vi "Load Test Data.vi"(8 "error in (no error)":errorcluster, 9 "To":timestamp, 10 "From":timestamp, 11 "Access in":refnum<class "Access.lvclass">) -> (0 "error out":errorcluster, 2 "Test Data Out":string[][](array[string]), 3 "Access out":refnum<class "Access.lvclass">)   [LabVIEW 2016, in "Database.lvlib" / "Access.lvclass"]
uses:
  Access.lvclass
  Access.lvclass/Access.ctl
  <vilib>/addons/database/Connection.llb/Conn Execute.vi
  <vilib>/addons/database/Recordset.llb/Rec Fetch Recordset Data (R).vi
  <vilib>/addons/database/Recordset.llb/Rec Destroy - Connection.vi
  <vilib>/addons/database/NI_Database_API.lvlib
  User Interface/User Interface.lvlib
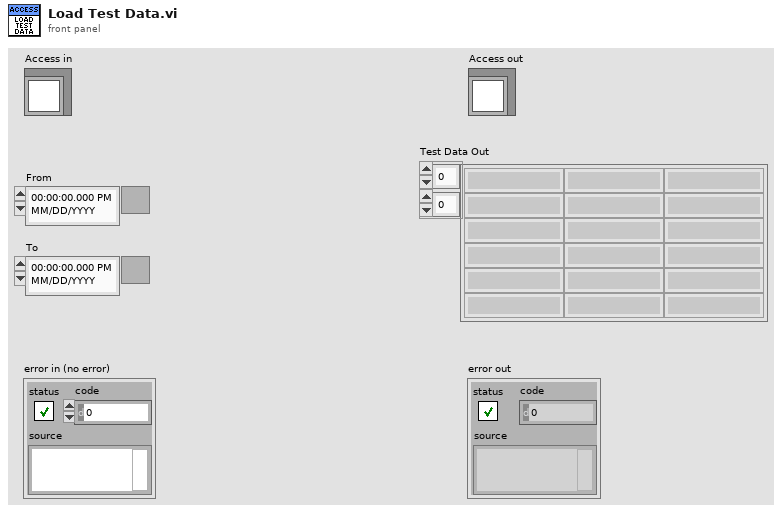
[diagram p1: front panel]
types:
  T1 = typedef "Database.lvlib/DB.lvclass/Column_info.ctl" = cluster{"Authentication":T2[], "Instr_Configuration":T2[], "Recipe":T2[], "Test_data":T2[]}
  T2 = typedef "NI_Database_API.lvlib/DB Tools Column Info.ctl" = cluster{"column name":string, "data type":T3, "size":i32, "allow null?":bool}
  T3 = typedef "NI_Database_API.lvlib/DB Tools DataTypes.ctl" = enum16{"String", "Long (I32)", "Single (SGL)", "Double (DBL)", "Date/Time", "Binary"}
  T4 = typedef "Database.lvlib/DB.lvclass/Table_info.ctl" = cluster{"Authentication":string, "Instr_Configuration":string, "Recipe":string, "Test_data":string}
  T5 = typedef "NI_Database_API.lvlib/Conn ObjectReference.ctl" = refnum<k1>
  T6 = typedef "NI_Database_API.lvlib/Rec ObjectReference.ctl" = refnum<k1>
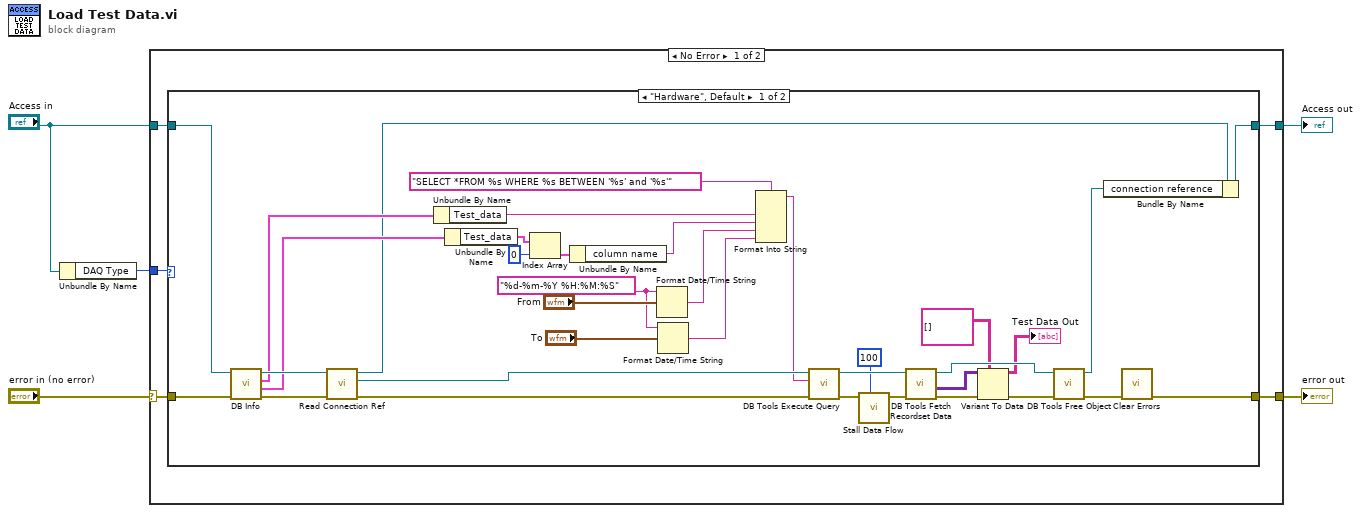
[diagram p0: block diagram]
diagram:
  n1 = Unbundle By Name("Access in") -> ("DAQ Type"=w1:enum16{"Hardware", "Simulation"})
  n2 = case shown="No Error" "error in (no error)" {
    selector: "error in (no error)" -> [w10 w48]
    tunnel: [w8 w49] -> w4
    tunnel: "Access in" -> [w9 w49]
    tunnel: [w7 w48] -> w3
    tunnel: w1 -> [w6 _]
    frame No Error {
      n3 = case shown="\"Hardware\", Default" w6 {
        tunnel: w10 -> [w45 w46]
        tunnel: w9 -> [w12 w47]
        tunnel: [w38 w47] -> w8
        tunnel: [w15 w46] -> w7
        frame "Hardware", Default {
          w21 = "%d-%m-%Y %H:%M:%S" ("time format string (%c)")
          n4 = call-dynamic "DB Info.vi"("error in (no error)"=w45, "Access in"=w12) -> ("error out"=w44:errorcluster, "Column_info"=w30:T1, "Table_info"=w33:T4, "Access out"=w43:refnum<class "Access.lvclass">)  [unwired: 6 in]
          n5 = call-dynamic "Read Connection Ref.vi"("error in (no error)"=w44, "Access in"=w43) -> ("error out"=w42:errorcluster, "connection reference"=w35:T5, "Access out"=w11:refnum<class "Access.lvclass">)  [unwired: 7 in]
          n6 = Unbundle By Name(w33) -> ("Test_data"=w31:string)
          n7 = Unbundle By Name(w30) -> ("Test_data"=w29:T2[])
          n8 = Index Array(array=w29, index=0) -> (element=w27:T2)
          n9 = Unbundle By Name(w27) -> ("column name"=w26:string)
          n10 = Format Date/Time String(time format string (%c)=w21, seconds (now)="From") -> (date/time string=w23:string)  [unwired: 1 in]
          n11 = Format Date/Time String(time format string (%c)=w21, seconds (now)="To") -> (date/time string=w22:string)  [unwired: 1 in]
          n12 = Format Into String(format string="SELECT *FROM %s WHERE %s BETWEEN '%s' and '%s'", w31, w26, w23, w22) -> (resulting string=w20:string)  [unwired: 2 in, 1 out]
          n13 = call-poly <vilib>:"DB Tools Execute Query.vi"("error in (no error)"=w42, "SQL query"=w20, "connection reference"=w35) -> ("error out"=w41:errorcluster, "recordset reference"=w37:T6)  [unwired: 5 in]
          n14 = call "Stall Data Flow.vi"("milliseconds to wait"=u32 100, "error in (no error)"=w41) -> ("error out"=w14:errorcluster)  [unwired: 9 in]
          n15 = call-poly <vilib>:"DB Tools Fetch Recordset Data.vi"("error in (no error)"=w14, "recordset reference"=w37) -> ("error out"=w40:errorcluster, "recordset data"=w17:variant[][], "recordset reference out"=w36:T6)  [unwired: 3 in]
          n16 = Variant To Data(error in=w40, type=string[][] [], Variant=w17) -> (data=→"Test Data Out":string[][], error out=w19:errorcluster)
          n17 = call-poly <vilib>:"DB Tools Free Object.vi"("error in (no error)"=w19, "recordset reference"=w36) -> ("error out"=w39:errorcluster, "connection reference"=w34:T5)  [unwired: 8 in]
          n18 = Bundle By Name(cluster=w11, "connection reference"=w34) -> (w38:refnum<class "Access.lvclass">)
          n19 = call <vilib>:"Clear Errors.vi"("error in (no error)"=w39) -> ("error out"=w15:errorcluster)  [unwired: 5 in, 1 out]
        }
        frame "Simulation" {
        }
      }
    }
    frame Error {
    }
  }
  "error out" <- w3
  "Access out" <- w4
